vi "validate.vi"(4 "output":sgl[][](array[numeric]), 5 "ptr":i64, 6 "error in (no error)":errorcluster, 7 "input":sgl[][](array[numeric])) -> (0 "prediction":sgl[][](array[numeric]), 1 "ptr out":i64, 2 "error out":errorcluster, 3 "error":sgl)   [LabVIEW 2016, in "CNet.lvlib"]
uses:
  CNet.lvlib
  Users/jg754/Documents/Visual Studio 2015/Projects/CLearn/x64/Release/CLearn.dll
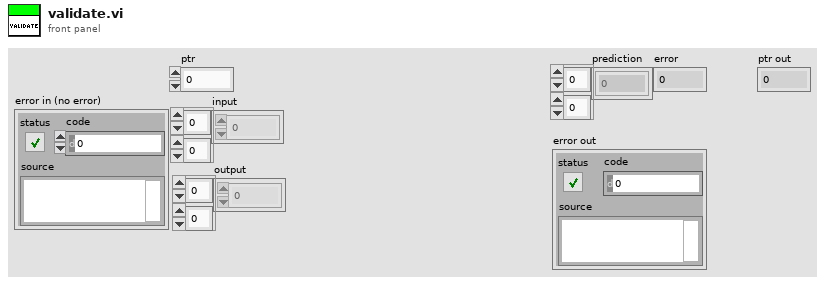
[diagram p1: front panel]
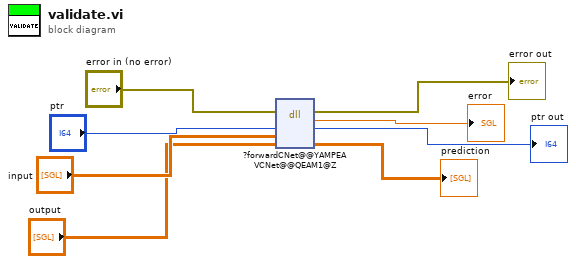
[diagram p0: block diagram]
diagram:
  n1 = dll-call lib="C:/Users/jg754/Documents/Visual Studio 2015/Projects/CLearn/x64/Release/CLearn.dll" fn="?forwardCNet@@YAMPEAVCNet@@QEAM1@Z"(error in="error in (no error)", "ptr"="ptr", "input"="input", "output"="output") -> (error out=→"error out":errorcluster, "error"=→"error":sgl, "ptr"=→"ptr out":i64, "output"=→"prediction":sgl[][])  [unwired: 3 in, 1 out]
